vi "start Julia ZMQ server v0.vi"(8 "error in (no error)":errorcluster, 11 "Julia ZMQ server file name":string="ZMQ-testserver.jl") -> (0 "error out":errorcluster, 3 "return code":i32)   [LabVIEW 2018, in "LV-Julia_ZMQ-Roundtrip_lib.lvlib"]
uses:
  LV-Julia_ZMQ-Roundtrip_lib.lvlib
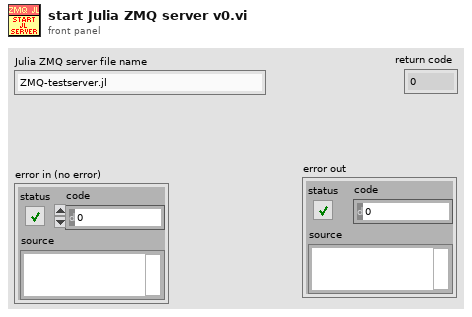
[diagram p1: front panel]
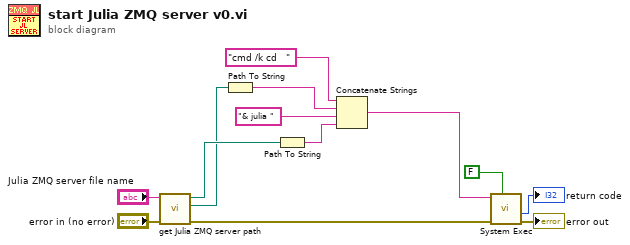
[diagram p0: block diagram]
diagram:
  n1 = call "get Julia ZMQ server path.vi"("error in (no error)"="error in (no error)", "Julia ZMQ server file name"="Julia ZMQ server file name") -> ("error out"=w11:errorcluster, "package base path"=w3:path, "Julia ZMQ server file path"=w8:path)  [unwired: 7 in]
  n2 = Path To String(path=w3) -> (string=w1:string)
  n3 = Path To String(path=w8) -> (string=w6:string)
  n4 = Concatenate Strings("cmd /k cd   ", w1, "& julia ", w6) -> (w5:string)
  n5 = call <vilib>:"System Exec.vi"("wait until completion? (T)"=FALSE, "error in (no error)"=w11, "command line"=w5) -> ("error out"=→"error out":errorcluster, "return code"=→"return code":i32)  [unwired: 5 in, 2 out]
